vi "DetecRecodManDlg.vi"(8 "error in":errorcluster) -> (0 "error out":errorcluster)   [LabVIEW 2014, in "ChaxuConfig.lvlib"]
uses:
  ChaxuConfig.lvlib
  DataBase/DataBase.lvlib
  DetectElecrodes/DetectElectros.lvlib
  CYY/cyy.lvlib
  Sample/Sample.lvlib
panel:
  in  "采样数据导出":bool
  in  "显示汇总信息":bool
  in  "显示所有采样信息":bool
  in  "退出":bool
  in  "选项卡控件":enum32{"采样信息", "区域采样信息汇总"}(tab)
  in  "按时间查询采样信息":i32(listbox)
  in  "终止时间":timestamp format="%<%Y-%m-%d %H:%M:%S>T"
  in  "起始时间":timestamp format="%<%Y-%m-%d %H:%M:%S>T"
  in  "查询":bool
  in  "删除按钮":bool
  in  "采样信息汇总":i32(listbox)
  out "采样信息总数":string
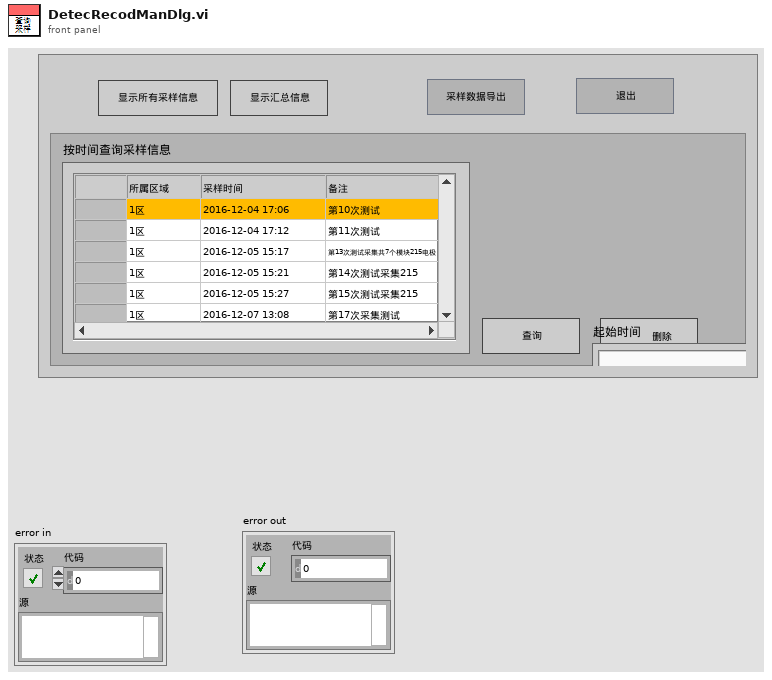
[diagram p1: front panel]
types:
  T1 = enum32{"invalid app kind", "Development System", "Run Time System", "Student Edition", "Embedded LabVIEW", "Evaluation", "Custom"}
  T2 = enum32{"Invalid", "Standard", "Closed", "Hidden", "Minimized", "Maximized"}
  T3 = cluster{"Core":cluster{"Current VI Reference":refnum<vi>, "Close Panel on Exit?":bool}, "Your Boolean data":bool, "Your string data":string, "终止时间 ":string, "起始时间":string, "SampleInfo":string[][], "sample_info_time":string, "SampleTime":string, "SampleAreaName":string}
  T4 = typedef "LVPoint32TypeDef.ctl" = cluster{"Horizontal":i32, "Vertical":i32}
  T5 = typedef "LVRowAndColumnTypeDef.ctl" = cluster{"Row":i32, "Column":i32}
  T6 = cluster{"Current VI Reference":refnum<vi>, "Close Panel on Exit?":bool}
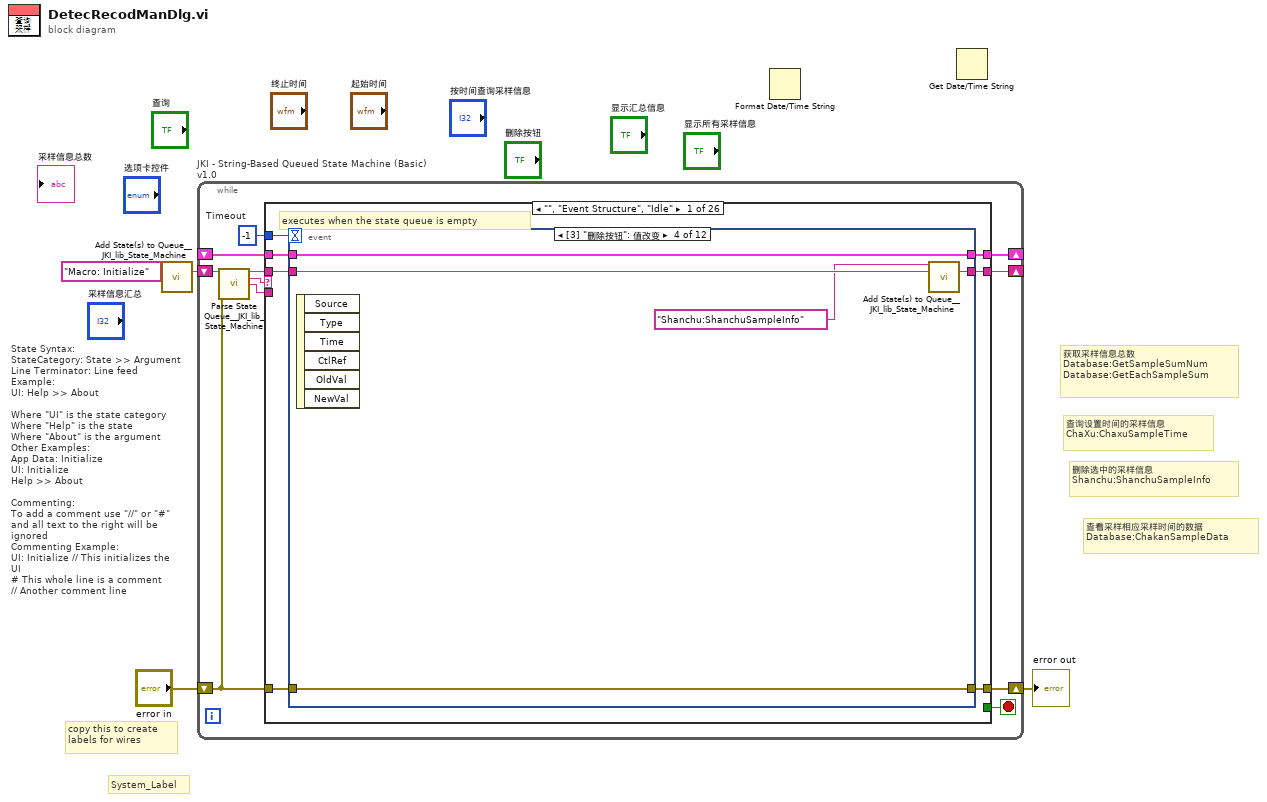
[diagram p0: block diagram]
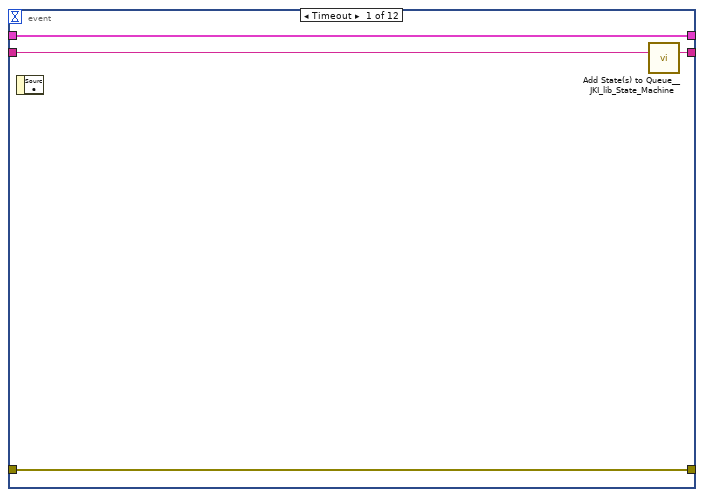
[diagram p2: hidden frame]
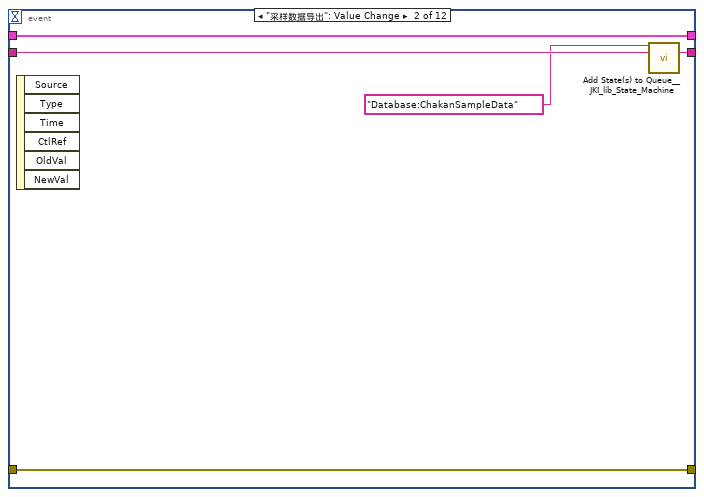
[diagram p3: hidden frame]
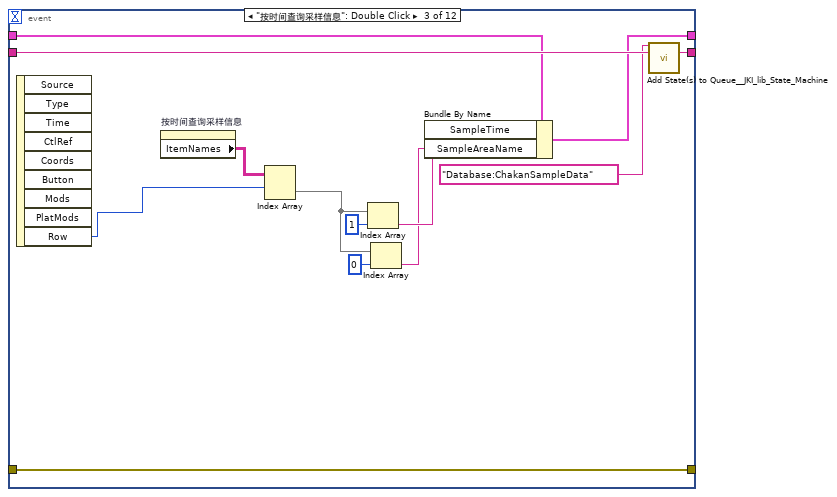
[diagram p4: hidden frame]
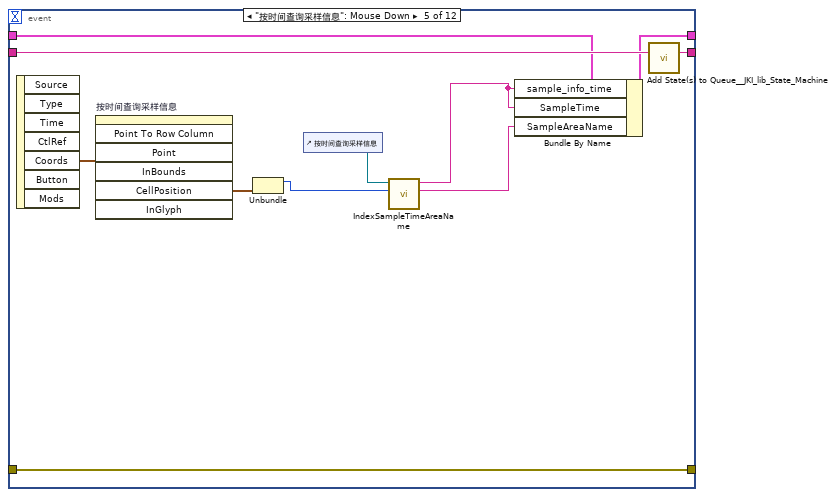
[diagram p5: hidden frame]
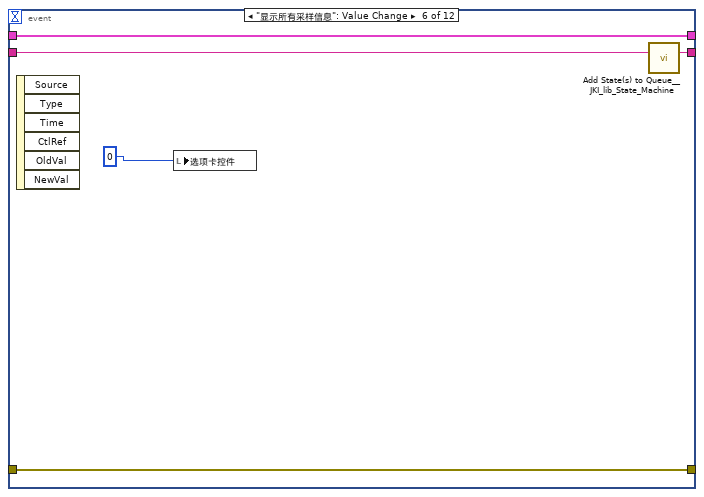
[diagram p6: hidden frame]
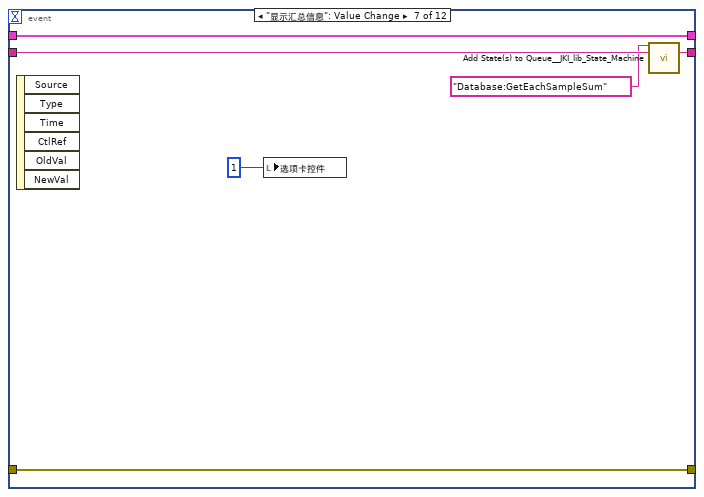
[diagram p7: hidden frame]
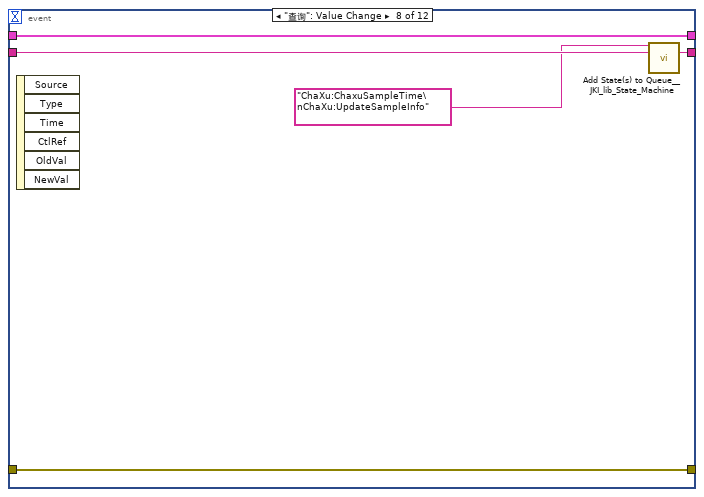
[diagram p8: hidden frame]
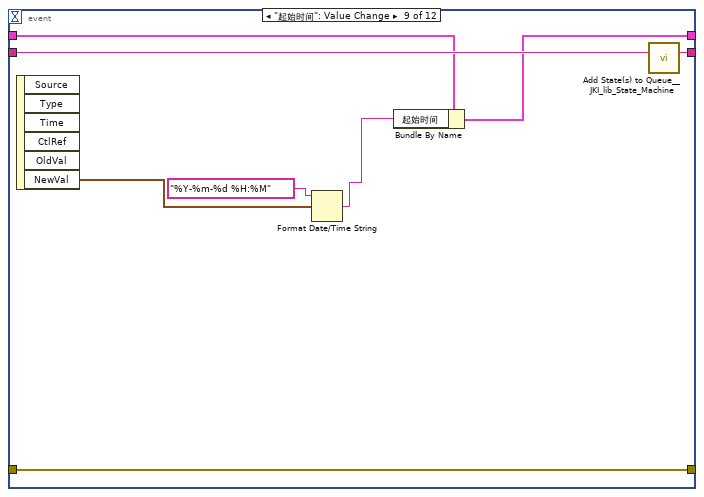
[diagram p9: hidden frame]
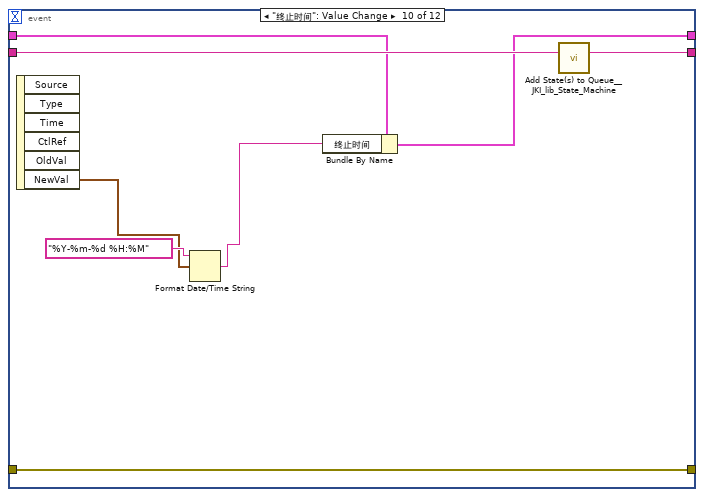
[diagram p10: hidden frame]
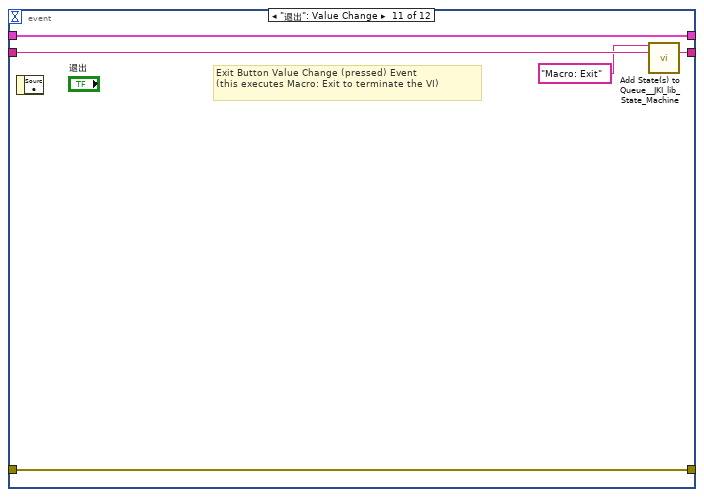
[diagram p11: hidden frame]
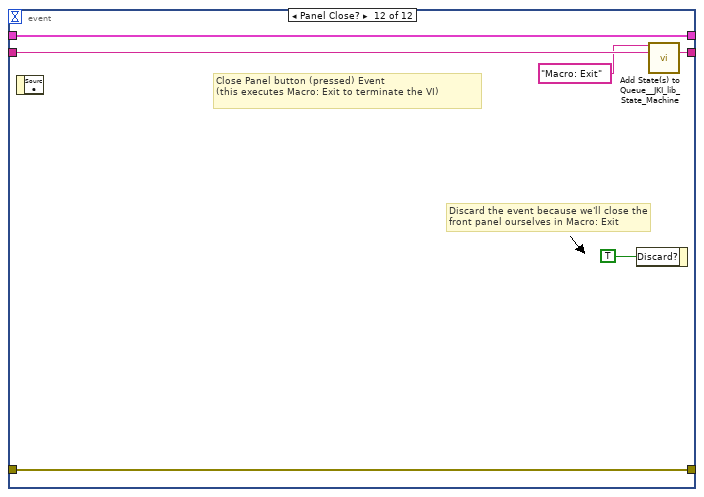
[diagram p12: hidden frame]
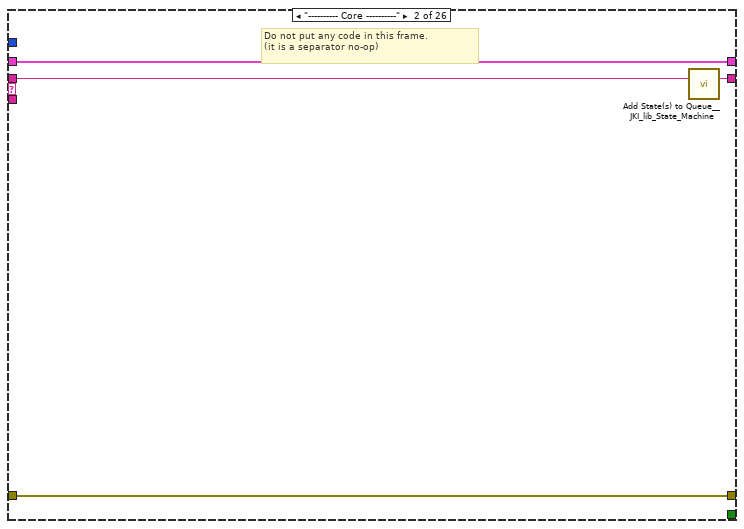
[diagram p13: hidden frame]
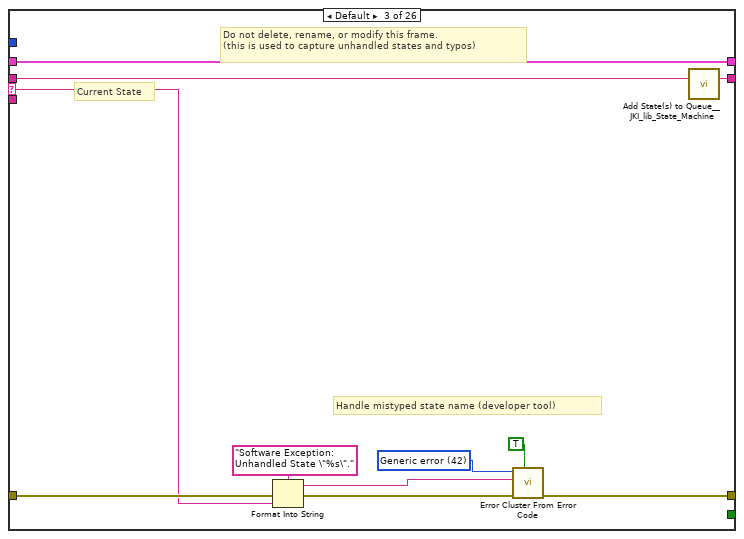
[diagram p14: hidden frame]
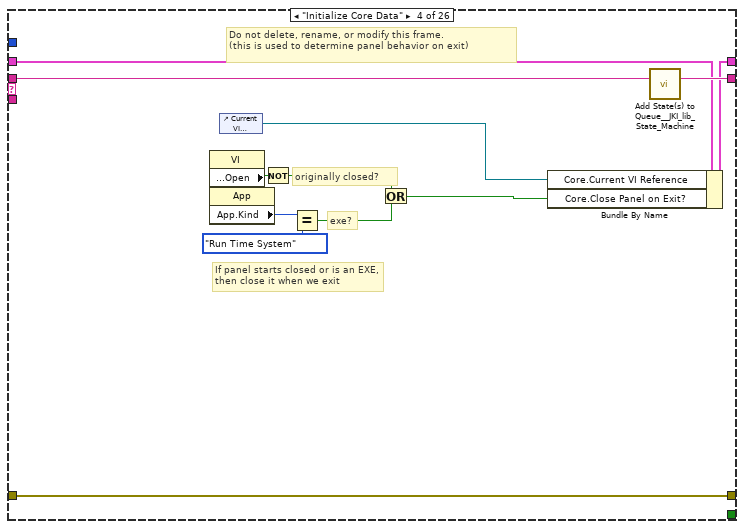
[diagram p15: hidden frame]
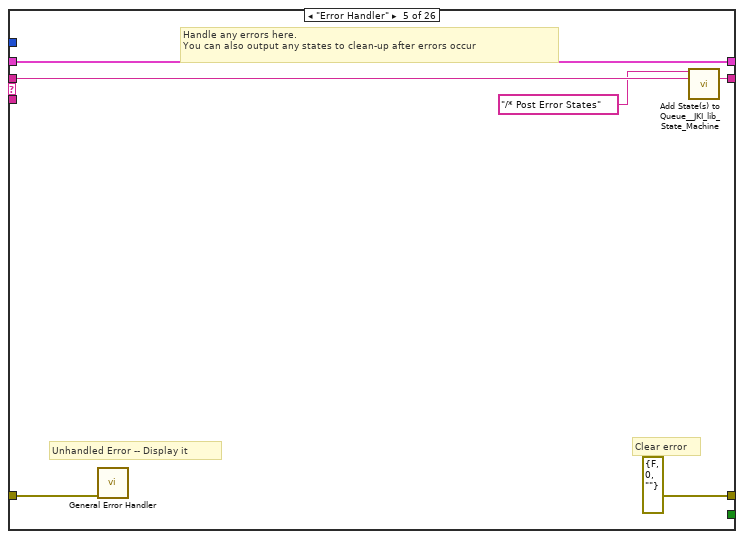
[diagram p16: hidden frame]
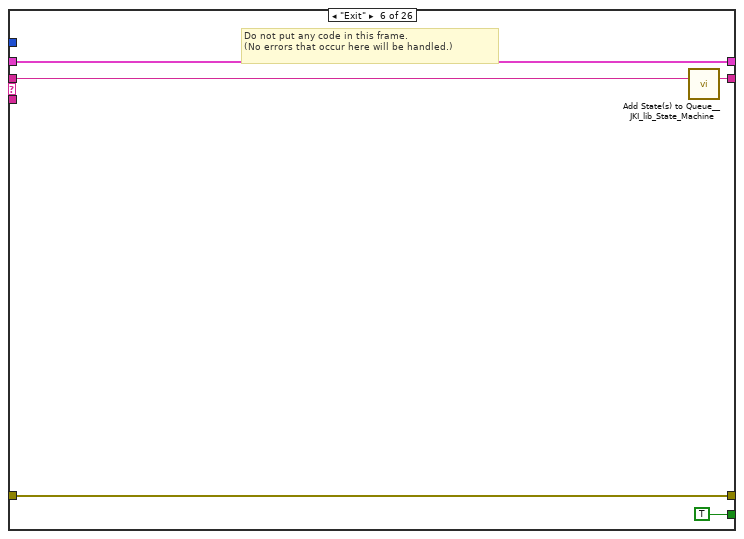
[diagram p17: hidden frame]
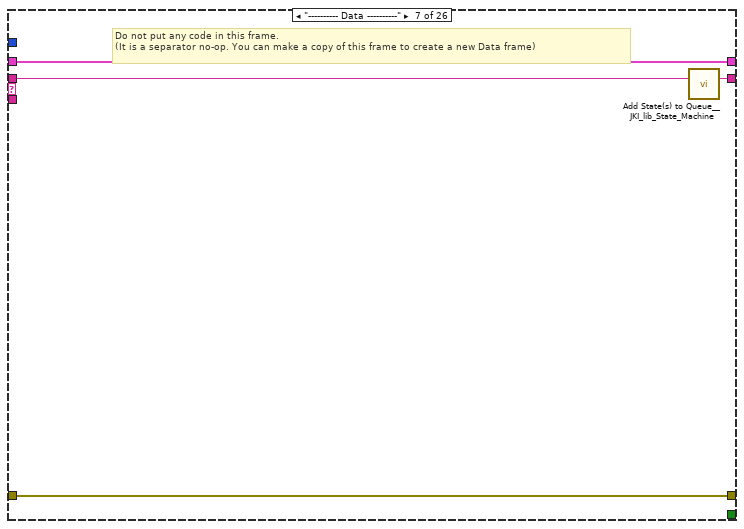
[diagram p18: hidden frame]
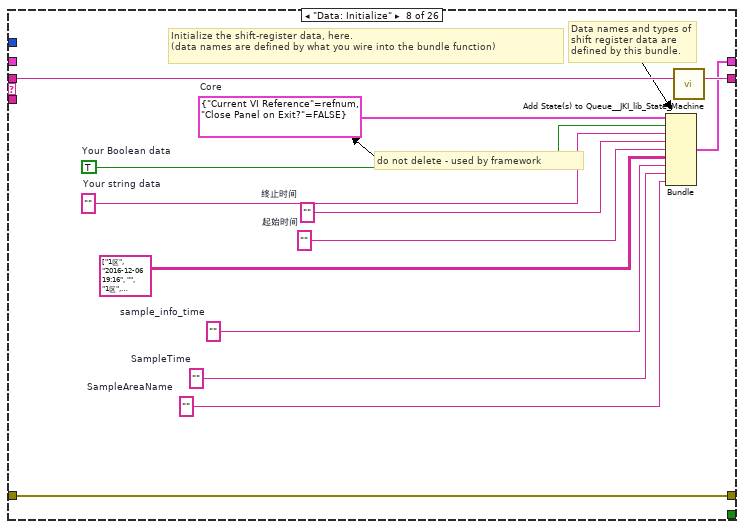
[diagram p19: hidden frame]
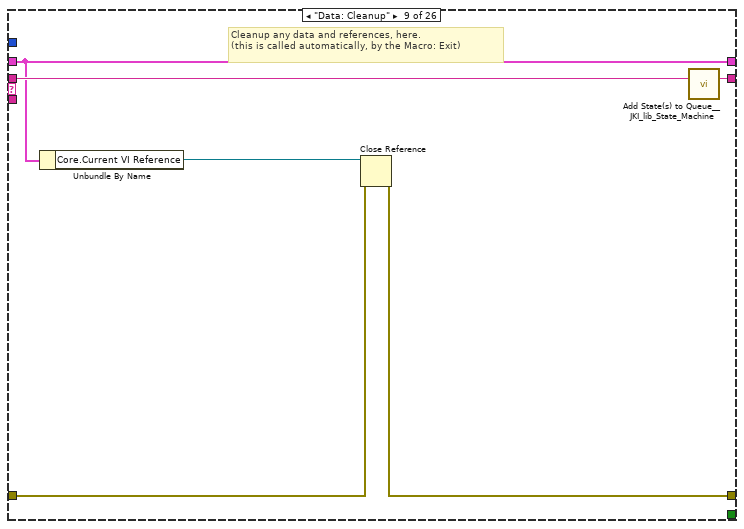
[diagram p20: hidden frame]
diagram:
  # "查看采样相应采样时间的数据\nDatabase:ChakanSampleData"
  # "删除选中的采样信息\nShanchu:ShanchuSampleInfo"
  # "查询设置时间的采样信息\nChaXu:ChaxuSampleTime"
  # "获取采样信息总数\nDatabase:GetSampleSumNum\nDatabase:GetEachSampleSum"
  # "State Syntax:\nStateCategory: State >> Argument\nLine Terminator: Line feed\nExample:\nUI: Help >> About\n\nWhere \"UI\" is the state category\nWhere \"Help\" is the state\nWhere \"About\" is the argument\nOther Examples:\nApp Data: Initialize\nUI: Initialize\nHelp >> About\n\nCommenting:\nTo add a comment use \"//\" or \"#\" and all text to the right will be ignored\nCommenting Example:\nUI: Initialize // This initializes the UI\n# This whole line is a comment\n// Another comment line"
  # "copy this to create labels for wires"
  # "System_Label"
  n1 = call <vilib>:"Add State(s) to Queue__JKI_lib_State_Machine.vi"("State(s) in (\"\")"="Macro: Initialize") -> ("States Out"=w4:string)  [unwired: 14 in]
  n2 = while "JKI - String-Based Queued State Machine (Basic) v1.0" {
    shift-right: [w8] -> _
    shift-left: _ -> [w7]
    shift-right: [w11] -> w2
    shift-left: "error in" -> [w5]
    shift-right: [w10] -> _
    shift-left: w4 -> [w12]
    stop <- w9 stop-if-true
    w6 = -1  # Timeout
    n3 = call <vilib>:"Parse State Queue__JKI_lib_State_Machine.vi"("State Queue"=w12, "Error In (no error)"=w5) -> ("Remaining States"=w14:string, "Current State"=w15:string, "Arguments"=w13:string)  [unwired: 11 in]
    n4 = case shown="\"\", \"Event Structure\", \"Idle\"" w15 {
      selector: w15 -> [_ _ w108 _ _ _ _ _ _ _ _ _ _ _ _ _ _ _ _ _ _ _ _ _ _ _]
      tunnel: w14 -> [w22 w107 w112 w130 w136 w141 w145 w158 w164 w168 w173 w179 w190 w216 w221 w231 w235 w239 w243 w255 w261 w278 w282 w290 w304 w316]
      tunnel: w13 -> [_ _ _ _ _ _ _ _ _ _ _ w174 w184 _ _ _ _ _ _ _ _ _ _ _ _ _]
      tunnel: w7 -> [w20 w104 w110 w121 w133 w139 w142 _ w159 w165 w171 w177 w186 w213 w218 w228 w232 w236 w240 w253 w259 w270 w279 w287 w302 w314]
      tunnel: [w19 w105 w114 w127 errorcluster {"status"=FALSE, "code"=0, "source"=""} ("error out") w138 w143 w155 w160 w166 w170 w175 w187 w214 w219 w229 w233 w237 w241 w250 w256 w276 w280 w288 w296 w311] -> w11
      tunnel: w5 -> [w18 w105 w113 w127 w132 w138 w143 w155 w161 w166 w170 w176 w188 w214 w219 w229 w233 w237 w241 w247 w257 w276 w280 w288 w297 w312]
      tunnel: [w21 w106 w111 w129 w135 w140 w144 w157 w163 w167 w172 w178 w189 w215 w220 w230 w234 w238 w242 w254 w260 w277 w281 w289 w303 w315] -> w10
      tunnel: [_ _ _ _ _ TRUE _ _ _ _ _ _ _ _ _ _ _ _ _ _ _ _ _ _ _ _] -> w9
      tunnel: [w17 w104 w110 w128 w133 w139 w142 w156 w159 w165 w171 w177 w186 w213 w218 w228 w232 w236 w240 w253 w259 w269 w279 w287 w302 w314] -> w8
      tunnel: w6 -> [w16 _ _ _ _ _ _ _ _ _ _ _ _ _ _ _ _ _ _ _ _ _ _ _ _ _]
      frame "", "Event Structure", "Idle" {
        # "executes when the state queue is empty"
        n5 = event shown="[3] \"删除按钮\": 值改变" {
          selector: _ -> [_ _ _ _ _ _ _ _ _ _ _ _]
          dyn-events: _ -> [_ _ _ _ _ _ _ _ _ _ _ _]
          timeout: w16 -> [_ _ _ _ _ _ _ _ _ _ _ _]
          tunnel: w22 -> [w26 w31 w44 w49 w60 w65 w71 w76 w84 w91 w97 w103]
          tunnel: [w25 w30 w43 w48 w59 w64 w70 w75 w83 w92 w96 w102] -> w21
          tunnel: w20 -> [w23 w28 w37 w46 w54 w62 w68 w73 w78 w86 w94 w100]
          tunnel: [w24 w29 w42 w47 w58 w63 w69 w74 w82 w90 w95 w101] -> w19
          tunnel: w18 -> [w24 w29 w42 w47 w58 w63 w69 w74 w82 w90 w95 w101]
          tunnel: [w23 w28 w36 w46 w53 w62 w68 w73 w77 w85 w94 w100] -> w17
          event Timeout {
            n6 = event-data() -> ()  [unwired: 1 in, 1 out]
            n7 = call <vilib>:"Add State(s) to Queue__JKI_lib_State_Machine.vi"("State(s) in (\"\")"=w26) -> ("States Out"=w25:string)  [unwired: 14 in]
          }
          event "采样数据导出": Value Change {
            n8 = event-data() -> ()  [unwired: 1 in, 6 out]
            n9 = call <vilib>:"Add State(s) to Queue__JKI_lib_State_Machine.vi"("State(s) in Front (\"\")"="Database:ChakanSampleData", "State(s) in (\"\")"=w31) -> ("States Out"=w30:string)  [unwired: 13 in]
          }
          event "按时间查询采样信息": Double Click {
            n10 = event-data() -> ("Row"=w40:i32)  [unwired: 1 in, 8 out]
            n11 = property on="按时间查询采样信息" class="MCListbox (严格)"() -> ("ItemNames"=w41:string[][])  [unwired: 2 in, 2 out]
            n12 = Index Array(array=w41, index (row)=w40) -> (element=w34:string[])  [unwired: 1 in]
            n13 = Index Array(array=w34, index=1 ("索引")) -> (element=w38:string)
            n14 = Index Array(array=w34, index=0 ("索引")) -> (element=w32:string)
            n15 = Bundle By Name(cluster=w37, "SampleTime"=w38, "SampleAreaName"=w32) -> (w36:T3)
            n16 = call <vilib>:"Add State(s) to Queue__JKI_lib_State_Machine.vi"("State(s) in Front (\"\")"="Database:ChakanSampleData", "State(s) in (\"\")"=w44) -> ("States Out"=w43:string)  [unwired: 13 in]
          }
          event "删除按钮": Value Change {
            n17 = event-data() -> ()  [unwired: 1 in, 6 out]
            n18 = call <vilib>:"Add State(s) to Queue__JKI_lib_State_Machine.vi"("State(s) in Front (\"\")"="Shanchu:ShanchuSampleInfo", "State(s) in (\"\")"=w49) -> ("States Out"=w48:string)  [unwired: 13 in]
          }
          event "按时间查询采样信息": Mouse Down {
            n19 = event-data() -> ("Coords"=w57:T4)  [unwired: 1 in, 6 out]
            n20 = invoke on="按时间查询采样信息" class="MCListbox (严格)" method="Point To Row Column"("Point"=w57) -> ("CellPosition"=w56:T5)  [unwired: 6 in, 6 out]
            n21 = Unbundle(w56) -> ("Row"=w55:i32)  [unwired: 1 out]
            n22 = control-ref of="按时间查询采样信息"() -> (w50:refnum<vi>)
            n23 = call "IndexSampleTimeAreaName.vi"("Row"=w55, "SampleInfo列表框"=w50) -> ("Area_name"=w51:string, "SampleTime"=w52:string)  [unwired: 8 in]
            n24 = Bundle By Name(cluster=w54, "sample_info_time"=w52, "SampleTime"=w52, "SampleAreaName"=w51) -> (w53:T3)
            n25 = call <vilib>:"Add State(s) to Queue__JKI_lib_State_Machine.vi"("State(s) in (\"\")"=w60) -> ("States Out"=w59:string)  [unwired: 14 in]
          }
          event "显示所有采样信息": Value Change {
            n26 = event-data() -> ()  [unwired: 1 in, 6 out]
            n27 = local write "选项卡控件"(0) -> ()
            n28 = call <vilib>:"Add State(s) to Queue__JKI_lib_State_Machine.vi"("State(s) in (\"\")"=w65) -> ("States Out"=w64:string)  [unwired: 14 in]
          }
          event "显示汇总信息": Value Change {
            n29 = event-data() -> ()  [unwired: 1 in, 6 out]
            n30 = local write "选项卡控件"(1) -> ()
            n31 = call <vilib>:"Add State(s) to Queue__JKI_lib_State_Machine.vi"("State(s) in Front (\"\")"="Database:GetEachSampleSum", "State(s) in (\"\")"=w71) -> ("States Out"=w70:string)  [unwired: 13 in]
          }
          event "查询": Value Change {
            n32 = event-data() -> ()  [unwired: 1 in, 6 out]
            n33 = call <vilib>:"Add State(s) to Queue__JKI_lib_State_Machine.vi"("State(s) in Front (\"\")"="ChaXu:ChaxuSampleTime\nChaXu:UpdateSampleInfo", "State(s) in (\"\")"=w76) -> ("States Out"=w75:string)  [unwired: 13 in]
          }
          event "起始时间": Value Change {
            n34 = event-data() -> ("NewVal"=w80:timestamp)  [unwired: 1 in, 5 out]
            n35 = Format Date/Time String(time format string (%c)="%Y-%m-%d %H:%M" ("时间格式字符串(%c)"), seconds (now)=w80) -> (date/time string=w79:string)  [unwired: 1 in]
            n36 = Bundle By Name(cluster=w78, "起始时间"=w79) -> (w77:T3)
            n37 = call <vilib>:"Add State(s) to Queue__JKI_lib_State_Machine.vi"("State(s) in (\"\")"=w84) -> ("States Out"=w83:string)  [unwired: 14 in]
          }
          event "终止时间": Value Change {
            n38 = event-data() -> ("NewVal"=w88:timestamp)  [unwired: 1 in, 5 out]
            n39 = Format Date/Time String(time format string (%c)="%Y-%m-%d %H:%M" ("时间格式字符串(%c)"), seconds (now)=w88) -> (date/time string=w87:string)  [unwired: 1 in]
            n40 = Bundle By Name(cluster=w86, "终止时间"=w87) -> (w85:T3)
            n41 = call <vilib>:"Add State(s) to Queue__JKI_lib_State_Machine.vi"("State(s) in (\"\")"=w91) -> ("States Out"=w92:string)  [unwired: 14 in]
          }
          event "退出": Value Change {
            # "Exit Button Value Change (pressed) Event\n(this executes Macro: Exit to terminate the VI)"
            n42 = event-data() -> ()  [unwired: 1 in, 1 out]
            n43 = call <vilib>:"Add State(s) to Queue__JKI_lib_State_Machine.vi"("State(s) in Front (\"\")"="Macro: Exit", "State(s) in (\"\")"=w97) -> ("States Out"=w96:string)  [unwired: 13 in]
          }
          event Panel Close? {
            # "Discard the event because we'll close the front panel ourselves in Macro: Exit"
            # "Close Panel button (pressed) Event\n(this executes Macro: Exit to terminate the VI)"
            n44 = event-data() -> ()  [unwired: 1 in, 1 out]
            n45 = event-data("Discard?"=TRUE) -> ()  [unwired: 1 in, 1 out]
            n46 = call <vilib>:"Add State(s) to Queue__JKI_lib_State_Machine.vi"("State(s) in Front (\"\")"="Macro: Exit", "State(s) in (\"\")"=w103) -> ("States Out"=w102:string)  [unwired: 13 in]
          }
        }
      }
      frame "---------- Core ----------" {
        # "Do not put any code in this frame.\n(it is a separator no-op)"
        n47 = call <vilib>:"Add State(s) to Queue__JKI_lib_State_Machine.vi"("State(s) in (\"\")"=w107) -> ("States Out"=w106:string)  [unwired: 14 in]
      }
      frame Default {
        w117 = 42 items=["No error", "Argument error", "Memory is full", "Out of zone", "End of file", "File already open", "Generic file I/O error", "File not found", "File permission error", "Disk is full", "Duplicate path", "Too many files open", "System feature not enabled", "Resource file not found", "Cannot add resource", "Resource not found", "Image not found", "Image memory error", "Pen does not exist", "Config type invalid", "Config token not found", "Config parse error", "Config memory error", "Bad external code format", "Bad external code offset", "External code not present", "Null window", "Destroy window error", "Null menu", "Print aborted", "Bad print record", "Print driver error", "Windows error during printing", "Memory error during printing", "Print dialog error", "Generic print error", "Invalid device refnum", "Device not found", "Device parameter error", "Device unit error", "Cannot open device", "Device call aborted", "Generic error", "Cancelled by user", "Object ID too low", "Object ID too high", "Object not in heap", "Unknown heap", "Unknown object (invalid DefProc)", "Unknown object (DefProc not in table)", "Message out of range", "Invalid (null) method", "Unknown message", "Manager call not supported", "Bad address", "Network operation in progress", "Network operation timed out", "Connection is busy", "Network attribute not supported", "Network error", "Address in use", "System out of memory", "Connection aborted", "Connection refused", "Not connected", "Already connected", "Connection closed", "Initialization error (interapplication manager)", "Bad occurrence", "Wait on unbound occurrence handler", "Occurrence queue overflow", "Datalog type conflict", "Unused", "Unrecognized type (interapplication manager)", "Memory corrupt", "Failed to make temporary DLL", "Old CIN version", "Drag socket not found", "Failed to load drop-object", "Failed to register OLE object", "Failed to release OLE object", "Format specifier type mismatch", "Unknown format specifier", "Too few format specifiers", "Too many format specifiers", "Scan failed", "Newer CIN version", "Error converting to variant", "Runtime menu error", "Password tampered", "Variant attribute not found", "Incompatible variant data type", "Event data is not available", "Event Store is not present", "Occurrence is not found", "Event Queue is not created", "Event info is not available", "Refnum passed is NULL", "Error retrieving Class GUID", "Error retrieving CoClass GUID", "Error retrieving TypeLib GUID.", "Bad built application magic bytes.", "Specific driver is different from the specific driver associated with the Logical Name.", "There is no session opened to the class driver.", "Max Error", "MAX - Error with config objects", "MAX - Error loading configuration", "MAX - Group not supported"]
        # "Current State"
        # "Do not delete, rename, or modify this frame.\n(this is used to capture unhandled states and typos)"
        # "Handle mistyped state name (developer tool)"
        n48 = Format Into String(format string="Software Exception: Unhandled State \"%s\"." ("message"), error in=w113, w108) -> (resulting string=w116:string, error out=w115:errorcluster)  [unwired: 1 in]
        n49 = call <vilib>:"Error Cluster From Error Code.vi"("show call chain? (False)"=TRUE, "error in (no error)"=w115, "error message (\"\")"=w116, "error code (0)"=w117) -> ("error out"=w114:errorcluster)  [unwired: 5 in]
        n50 = call <vilib>:"Add State(s) to Queue__JKI_lib_State_Machine.vi"("State(s) in (\"\")"=w112) -> ("States Out"=w111:string)  [unwired: 14 in]
      }
      frame "Initialize Core Data" {
        # "Do not delete, rename, or modify this frame.\n(this is used to determine panel behavior on exit)"
        # "originally closed?"
        # "exe?"
        # "If panel starts closed or is an EXE, then close it when we exit"
        n51 = property class="VI"() -> ("Front Panel.Open"=w126:bool)  [unwired: 2 in, 2 out]
        n52 = property class="App"() -> ("App.Kind"=w125:T1)  [unwired: 2 in, 2 out]
        n53 = control-ref of="Current VI Reference"() -> (w119:refnum<vi>)
        n54 = Not(x=w126) -> (.not. x?=w123:bool)
        n55 = Equal?(x=w125, y=T1."Run Time System" ("Application:Kind")) -> (x = y?=w122:bool)
        n56 = Or(x=w123, y=w122) -> (x .or. y?=w120:bool)
        n57 = Bundle By Name(cluster=w121, "Core.Current VI Reference"=w119, "Core.Close Panel on Exit?"=w120) -> (w128:T3)
        n58 = call <vilib>:"Add State(s) to Queue__JKI_lib_State_Machine.vi"("State(s) in (\"\")"=w130) -> ("States Out"=w129:string)  [unwired: 14 in]
      }
      frame "Error Handler" {
        # "Unhandled Error -- Display it"
        # "Handle any errors here.\nYou can also output any states to clean-up after errors occur"
        # "Clear error"
        n59 = call <vilib>:"General Error Handler.vi"("error in (no error)"=w132) -> ()  [unwired: 10 in, 5 out]
        n60 = call <vilib>:"Add State(s) to Queue__JKI_lib_State_Machine.vi"("State(s) in Front (\"\")"="/* Post Error States", "State(s) in (\"\")"=w136) -> ("States Out"=w135:string)  [unwired: 13 in]
      }
      frame "Exit" {
        # "Do not put any code in this frame.\n(No errors that occur here will be handled.)"
        n61 = call <vilib>:"Add State(s) to Queue__JKI_lib_State_Machine.vi"("State(s) in (\"\")"=w141) -> ("States Out"=w140:string)  [unwired: 14 in]
      }
      frame "---------- Data ----------" {
        # "Do not put any code in this frame.\n(It is a separator no-op. You can make a copy of this frame to create a new Data frame)"
        n62 = call <vilib>:"Add State(s) to Queue__JKI_lib_State_Machine.vi"("State(s) in (\"\")"=w145) -> ("States Out"=w144:string)  [unwired: 14 in]
      }
      frame "Data: Initialize" {
        w146 = ""  # SampleAreaName
        w147 = ""  # SampleTime
        w148 = ""  # sample_info_time
        w150 = ""  # 起始时间
        w151 = ""  # 终止时间
        w152 = T6 {"Current VI Reference"=refnum, "Close Panel on Exit?"=FALSE}  # Core
        w154 = TRUE  # Your Boolean data
        w153 = ""  # Your string data
        # "do not delete - used by framework"
        # "Data names and types of shift register data are defined by this bundle."
        # "Initialize the shift-register data, here.\n(data names are defined by what you wire into the bundle function)"
        n63 = Bundle("Core"=w152, "Your Boolean data"=w154, "Your string data"=w153, "终止时间"=w151, "起始时间"=w150, "SampleInfo"=string[][] [["1区", "2016-12-06 19:16", ""], ["1区", "2016-12-07 13:08", "第17次采集测试"]], "sample_info_time"=w148, "SampleTime"=w147, "SampleAreaName"=w146) -> (w156:T3)  [unwired: 1 in]
        n64 = call <vilib>:"Add State(s) to Queue__JKI_lib_State_Machine.vi"("State(s) in (\"\")"=w158) -> ("States Out"=w157:string)  [unwired: 14 in]
      }
      frame "Data: Cleanup" {
        # "Cleanup any data and references, here.\n(this is called automatically, by the Macro: Exit)"
        n65 = Unbundle By Name(w159) -> ("Core.Current VI Reference"=w162:refnum<vi>)
        n66 = Close Reference(reference=w162, error in (no error)=w161) -> (error out=w160:errorcluster)
        n67 = call <vilib>:"Add State(s) to Queue__JKI_lib_State_Machine.vi"("State(s) in (\"\")"=w164) -> ("States Out"=w163:string)  [unwired: 14 in]
      }
      frame "---------- UI ----------" {
        # "Do not put any code in this frame.\n(It is a separator no-op. You can make a copy of this frame to create a new UI frame)"
        n68 = call <vilib>:"Add State(s) to Queue__JKI_lib_State_Machine.vi"("State(s) in (\"\")"=w168) -> ("States Out"=w167:string)  [unwired: 14 in]
      }
      frame "UI: Initialize" {
        # "Initialize the User Interface, here.\n(this is called automatically, by the Macro: Init)"
        n69 = call <vilib>:"Add State(s) to Queue__JKI_lib_State_Machine.vi"("State(s) in Front (\"\")"="Database:GetSampleSumNum\nDatabase:GetEachSampleSum", "State(s) in (\"\")"=w173) -> ("States Out"=w172:string)  [unwired: 13 in]
      }
      frame "UI: Cursor Set" {
        # "Argument"
        # "Set and Unset Cursor Busy.\n(Usage: \"UI: Cursor Set >> Busy|Idle\")"
        n70 = case shown="\"Idle\", 默认" w174 {
          tunnel: w176 -> [w181 w183]
          tunnel: [w180 w182] -> w175
          frame "Idle", Default {
            n71 = call <vilib>:"Unset Busy.vi"("error in (no error)"=w181) -> ("error out"=w180:errorcluster)  [unwired: 10 in]
          }
          frame "Busy" {
            n72 = call <vilib>:"Set Busy.vi"("error in (no error)"=w183) -> ("error out"=w182:errorcluster)  [unwired: 9 in, 1 out]
          }
        }
        n73 = call <vilib>:"Add State(s) to Queue__JKI_lib_State_Machine.vi"("State(s) in (\"\")"=w179) -> ("States Out"=w178:string)  [unwired: 14 in]
      }
      frame "UI: Front Panel State" {
        # "Argument"
        # "Set Front Panel Open or Closed\n(Usage: \"UI: Front Panel State >> Open|Close\")"
        n74 = Unbundle By Name(w186) -> ("Core.Current VI Reference"=w185:refnum<vi>)
        n75 = case shown="\"Open\", 默认" w184 {
          tunnel: w188 -> [w194 w207]
          tunnel: [w196 w208] -> w187
          tunnel: w185 -> [w195 w205]
          frame "Open", Default {
            n76 = property class="VI"(reference=w195, error in=w194) -> (reference out=w192:refnum<vi>, error out=w193:errorcluster, "Front Panel.Open"=w191:bool)
            n77 = case shown="假" w191 {
              tunnel: [w199 w202] -> w196
              tunnel: w193 -> [w198 w202]
              tunnel: w192 -> [w197 _]
              frame False {
                n78 = invoke class="VI" method="FP.Open"(reference=w197, error in=w198, "Activate"=TRUE, "State"=T2."Standard") -> (error out=w199:errorcluster)  [unwired: 1 in, 4 out]
              }
              frame True {
              }
            }
          }
          frame "Close" {
            n79 = property class="VI"(reference=w205, error in=w207) -> (reference out=w204:refnum<vi>, error out=w206:errorcluster, "Front Panel.Open"=w203:bool)
            n80 = case shown="真" w203 {
              tunnel: [w209 w212] -> w208
              tunnel: w206 -> [w209 w211]
              tunnel: w204 -> [_ w210]
              frame False {
              }
              frame True {
                n81 = invoke class="VI" method="FP.Close"(reference=w210, error in=w211) -> (error out=w212:errorcluster)  [unwired: 1 in, 2 out]
              }
            }
          }
        }
        n82 = call <vilib>:"Add State(s) to Queue__JKI_lib_State_Machine.vi"("State(s) in (\"\")"=w190) -> ("States Out"=w189:string)  [unwired: 14 in]
      }
      frame "---------- Macro ----------" {
        # "Do not put any code in this frame.\n(It is a separator no-op. You can make a copy of this frame to create a new Macro frame)"
        n83 = call <vilib>:"Add State(s) to Queue__JKI_lib_State_Machine.vi"("State(s) in (\"\")"=w216) -> ("States Out"=w215:string)  [unwired: 14 in]
      }
      frame "Macro: Initialize" {
        w217 = "Data: Initialize\nInitialize Core Data\nUI: Initialize\nUI: Front Panel State >> Open"  # Data: Initialize Initialize Core Data UI: Initialize UI: Front Panel State >> Open
        # "Initialization Macro\n(This is called once, when the VI starts)"
        n84 = call <vilib>:"Add State(s) to Queue__JKI_lib_State_Machine.vi"("State(s) in Front (\"\")"=w217, "State(s) in (\"\")"=w221) -> ("States Out"=w220:string)  [unwired: 13 in]
      }
      frame "Macro: Exit" {
        # "Exit Macro\n(This is called once, when the VI exits)"
        n85 = Unbundle By Name(w228) -> ("Core.Close Panel on Exit?"=w227:bool)
        n86 = Select(t="UI: Front Panel State >> Close", s=w227, f="") -> (s? t:f=w224:string)
        n87 = call <vilib>:"Add State(s) to Queue__JKI_lib_State_Machine.vi"("State(s) in (\"\")"=w224, "State(s) at Back (\"\")"="Data: Cleanup\nExit") -> ("States Out"=w222:string)  [unwired: 13 in]
        n88 = call <vilib>:"Add State(s) to Queue__JKI_lib_State_Machine.vi"("State(s) in Front (\"\")"=w222, "State(s) in (\"\")"=w231) -> ("States Out"=w230:string)  [unwired: 13 in]
      }
      frame "---------- New Category ----------" {
        # "Template Separator\n(You can make a copy of, or modify, this frame)"
        n89 = call <vilib>:"Add State(s) to Queue__JKI_lib_State_Machine.vi"("State(s) in (\"\")"=w235) -> ("States Out"=w234:string)  [unwired: 14 in]
      }
      frame "New Category: 1" {
        # "Your code here.\n(You can make a copy of, or modify, this frame)"
        n90 = call <vilib>:"Add State(s) to Queue__JKI_lib_State_Machine.vi"("State(s) in (\"\")"=w239) -> ("States Out"=w238:string)  [unwired: 14 in]
      }
      frame "New Category: 2" {
        # "Your code here.\n(You can make a copy of, or modify, this frame)"
        n91 = call <vilib>:"Add State(s) to Queue__JKI_lib_State_Machine.vi"("State(s) in (\"\")"=w243) -> ("States Out"=w242:string)  [unwired: 14 in]
      }
      frame "Shanchu:ShanchuSampleInfo" {
        # "delete from t_sample_info where sample_info_time='%s';"
        # "Your code here.\n(You can make a copy of, or modify, this frame)"
        n92 = Unbundle By Name(w253) -> ("sample_info_time"=w245:string)
        n93 = Format Into String(format string="delete from t_test_data where sample_info_time='%s';", w245) -> (resulting string=w248:string)  [unwired: 2 in, 1 out]
        n94 = Format Into String(format string="delete from t_sample_info where sample_info_time='%s';", w245) -> (resulting string=w251:string)  [unwired: 2 in, 1 out]
        n95 = call "deleteData.vi"("error in"=w247, "SQL query"=w248) -> ("error out"=w246:errorcluster)  [unwired: 9 in]
        n96 = call "deleteData.vi"("error in"=w246, "SQL query"=w251) -> ("error out"=w250:errorcluster)  [unwired: 9 in]
        n97 = call <vilib>:"Add State(s) to Queue__JKI_lib_State_Machine.vi"("State(s) in Front (\"\")"="ChaXu:ChaxuSampleTime\nChaXu:UpdateSampleInfo", "State(s) in (\"\")"=w255) -> ("States Out"=w254:string)  [unwired: 13 in]
      }
      frame "ChaXu:UpdateSampleInfo" {
        (unwired) string[] ["所属区域", "采样时间", "备注"]
        # "Your code here.\n(You can make a copy of, or modify, this frame)"
        n98 = Unbundle By Name(w259) -> ("SampleInfo"=w258:string[][])
        n99 = property on="按时间查询采样信息" class="MCListbox (严格)"(error in=w257, "ItemNames"=w258) -> (error out=w256:errorcluster)  [unwired: 1 in, 1 out]
        n100 = call <vilib>:"Add State(s) to Queue__JKI_lib_State_Machine.vi"("State(s) in (\"\")"=w261) -> ("States Out"=w260:string)  [unwired: 14 in]
      }
      frame "ChaXu:ChaxuSampleTime" {
        # "Your code here.\n(You can make a copy of, or modify, this frame)"
        n101 = Unbundle By Name(w270) -> ()  [unwired: 1 out]
        n102 = Unbundle By Name(w270) -> ()  [unwired: 1 out]
        n103 = local read "起始时间"() -> (w265:timestamp)
        n104 = local read "终止时间"() -> (w263:timestamp)
        n105 = Format Date/Time String(time format string (%c)="%Y-%m-%d %H:%M" ("时间格式字符串(%c)"), seconds (now)=w263) -> (date/time string=w262:string)  [unwired: 1 in]
        n106 = Format Date/Time String(time format string (%c)="%Y-%m-%d %H:%M" ("时间格式字符串(%c)"), seconds (now)=w265) -> (date/time string=w266:string)  [unwired: 1 in]
        n107 = Format Into String(format string="select area_name,sample_info_time,sample_info_desc from t_sample_info\nwhere sample_info_time>='%s' and sample_info_time <='%s';", w266, w262) -> (resulting string=w275:string)  [unwired: 2 in, 1 out]
        n108 = call "SelectData.vi"("SQL query"=w275) -> ("recordset data"=w274:variant[][])  [unwired: 7 in, 1 out]
        n109 = call "ReadDataFromDatabase.vi"("长度"=3, "index"=0, "recordset data"=w274) -> ("所有记录"=w271:string[][])  [unwired: 7 in, 1 out]
        n110 = Bundle By Name(cluster=w270, "SampleInfo"=w271) -> (w269:T3)
        n111 = call <vilib>:"Add State(s) to Queue__JKI_lib_State_Machine.vi"("State(s) in (\"\")"=w278) -> ("States Out"=w277:string)  [unwired: 14 in]
      }
      frame "----------Database---------" {
        # "Your code here.\n(You can make a copy of, or modify, this frame)"
        n112 = call <vilib>:"Add State(s) to Queue__JKI_lib_State_Machine.vi"("State(s) in (\"\")"=w282) -> ("States Out"=w281:string)  [unwired: 14 in]
      }
      frame "Database:ChakanSampleData" {
        n113 = Unbundle By Name(w287) -> ("SampleTime"=w284:string, "SampleAreaName"=w283:string)
        n114 = call "GetSampleData.vi"("SampleInfoTime"=w284) -> ("是否存在记录"=w286:bool, "所有记录"=w285:string[][])  [unwired: 7 in, 2 out]
        n115 = case shown="真" w286 {
          tunnel: w285 -> [_ w292]
          tunnel: w284 -> [_ w294]
          tunnel: w283 -> [_ w293]
          frame False {
            n116 = One Button Dialog(message="此时间无采样数据，请从新查询" ("消息")) -> ()  [unwired: 1 in, 1 out]
          }
          frame True {
            n117 = call "SampleDataDlg.vi"("采样数据in"=w292, "采样区域in"=w293, "采样时间in"=w294) -> ()  [unwired: 8 in, 1 out]
          }
        }
        n118 = call <vilib>:"Add State(s) to Queue__JKI_lib_State_Machine.vi"("State(s) in (\"\")"=w290) -> ("States Out"=w289:string)  [unwired: 14 in]
      }
      frame "Database:GetEachSampleSum" {
        # "Your code here.\n(You can make a copy of, or modify, this frame)"
        n119 = call "SelectData.vi"("SQL query"="SELECT area_name,count(*)sumnum ,sample_info_time \nFROM t_sample_info group by area_name;", "error in"=w297) -> ("recordset data"=w300:variant[][], "error out"=w296:errorcluster)  [unwired: 6 in]
        n120 = call "ReadDataFromDatabase.vi"("长度"=3, "index"=0, "recordset data"=w300) -> ("所有记录"=w295:string[][])  [unwired: 7 in, 1 out]
        n121 = property on="采样信息汇总" class="MCListbox (严格)"("ItemNames"=w295) -> ()  [unwired: 2 in, 2 out]
        n122 = call <vilib>:"Add State(s) to Queue__JKI_lib_State_Machine.vi"("State(s) in (\"\")"=w304) -> ("States Out"=w303:string)  [unwired: 14 in]
      }
      frame "Database:GetSampleSumNum" {
        # "Your code here.\n(You can make a copy of, or modify, this frame)"
        n123 = call "SelectData.vi"("SQL query"="select count(*) from t_sample_info;", "error in"=w312) -> ("recordset data"=w310:variant[][], "error out"=w311:errorcluster)  [unwired: 6 in]
        n124 = call "ReadDataFromDatabase.vi"("长度"=1, "index"=0, "recordset data"=w310) -> ("一行记录"=w307:string[])  [unwired: 7 in, 1 out]
        n125 = Index Array(array=w307, index=0 ("索引")) -> (element=w305:string)
        n126 = local write "采样信息总数"(w305) -> ()
        n127 = call <vilib>:"Add State(s) to Queue__JKI_lib_State_Machine.vi"("State(s) in (\"\")"=w316) -> ("States Out"=w315:string)  [unwired: 14 in]
      }
    }
  }
  "error out" <- w2
  n128 = Format Date/Time String() -> ()  [unwired: 3 in, 1 out]
  n129 = Get Date/Time String() -> ()  [unwired: 3 in, 2 out]
